vi "Write Excel File.vi"   [LabVIEW 2023]
doc: "Demonstrates how to create a .xlsx file with the Write To Measurement File Express VI. A .xlsx file can be opened in Microsoft Excel 2007 or later. Running this example does not require Microsoft Excel to be installed on this computer."
panel:
  # "Overview: Demonstrates how to create a .xlsx file with the Write To Measurement File Express VI that can be opened in Microsoft Excel.\nInstructions:\n1. Run the VI. It will create a .xlsx file located at [LabVIEW Data]\\Example Excel File.xlsx.\n2. Open the file in Microsoft Excel 2007 or later. It should contain 100 sets of Sine data.\n3. Delete the .xlsx file when you are done.\n\nNote: Running this VI does not require Microsoft Excel to be installed on this computer."
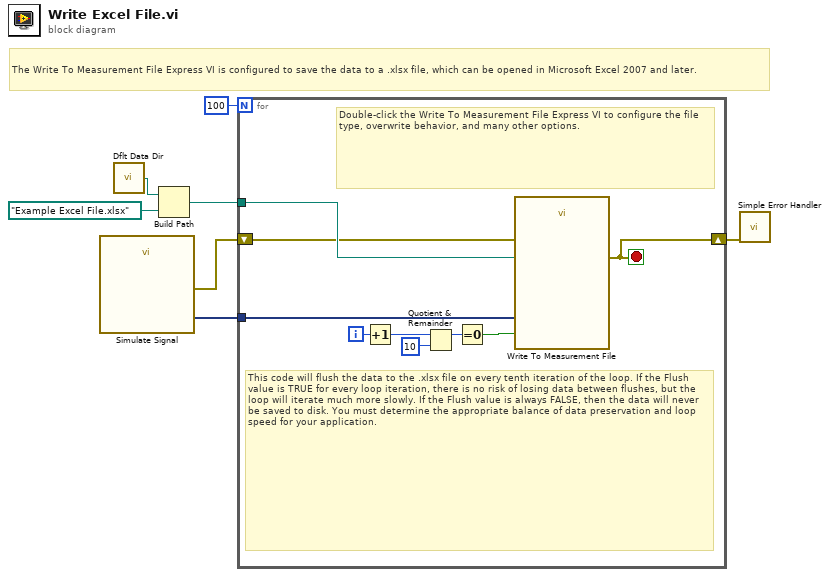
[diagram p0: block diagram]
diagram:
  # "The Write To Measurement File Express VI is configured to save the data to a .xlsx file, which can be opened in Microsoft Excel 2007 and later."
  n1 = call "Simulate Signal"() -> ("Sine"=w5:dynamicdata, "error out"=w7:errorcluster)  [unwired: 14 in]
  n2 = call <vilib>:"Dflt Data Dir.vi"() -> ("App:Default Data Directory"=w3:path)
  n3 = Build Path(base path=w3, name or relative path=path "Example Excel File.xlsx" ("default name")) -> (appended path=w1:path)
  n4 = for {
    N: 100 -> [_]
    tunnel: w5 -> [w16]
    shift-right: [w9] -> w6
    shift-left: w7 -> [w14]
    tunnel: w1 -> [w15]
    i -> [w13]
    stop <- w9 stop-if-true
    # "Double-click the Write To Measurement File Express VI to configure the file type, overwrite behavior, and many other options."
    # "This code will flush the data to the .xlsx file on every tenth iteration of the loop. If the Flush value is TRUE for every loop iteration, there is no risk of losing data between flushes, but the loop will iterate much more slowly. If the Flush value is always FALSE, then the data will never be saved to disk. You must determine the appropriate balance of data preservation and loop speed for your application."
    n5 = Increment(x=w13) -> (x+1=w10:i32)
    n6 = Quotient & Remainder(x=w10, y=10) -> (x-y*floor(x/y)=w12:i32)  [unwired: 1 out]
    n7 = Equal To 0?(x=w12) -> (x = 0?=w8:bool)
    n8 = call "Write To Measurement File"("Signals"=w16, "Flush? (T)"=w8, "error in (no error)"=w14, "Filename"=w15) -> ("error out"=w9:errorcluster)  [unwired: 13 in, 2 out]
  }
  n9 = call <vilib>:"Simple Error Handler.vi"("error in (no error)"=w6) -> ()  [unwired: 4 in, 5 out]
